vi "Example png string to imaq image.vi"() -> ()   [LabVIEW 2020]
uses:
  <vilib>/vision/Image Controls.llb/IMAQ Image.ctl
  <vilib>/wsapi/NI_WebServices.lvlib
  <vilib>/vision/NI_Vision_Development_Module.lvlib
panel:
  out "Image 2":T1(plugin-control)
  out "error out 2":errorcluster
  in  "error in (no error)":errorcluster
  out "Image Out":T1
  in  "File Path":path
  out "Image":T1(plugin-control)
  in  "String":string
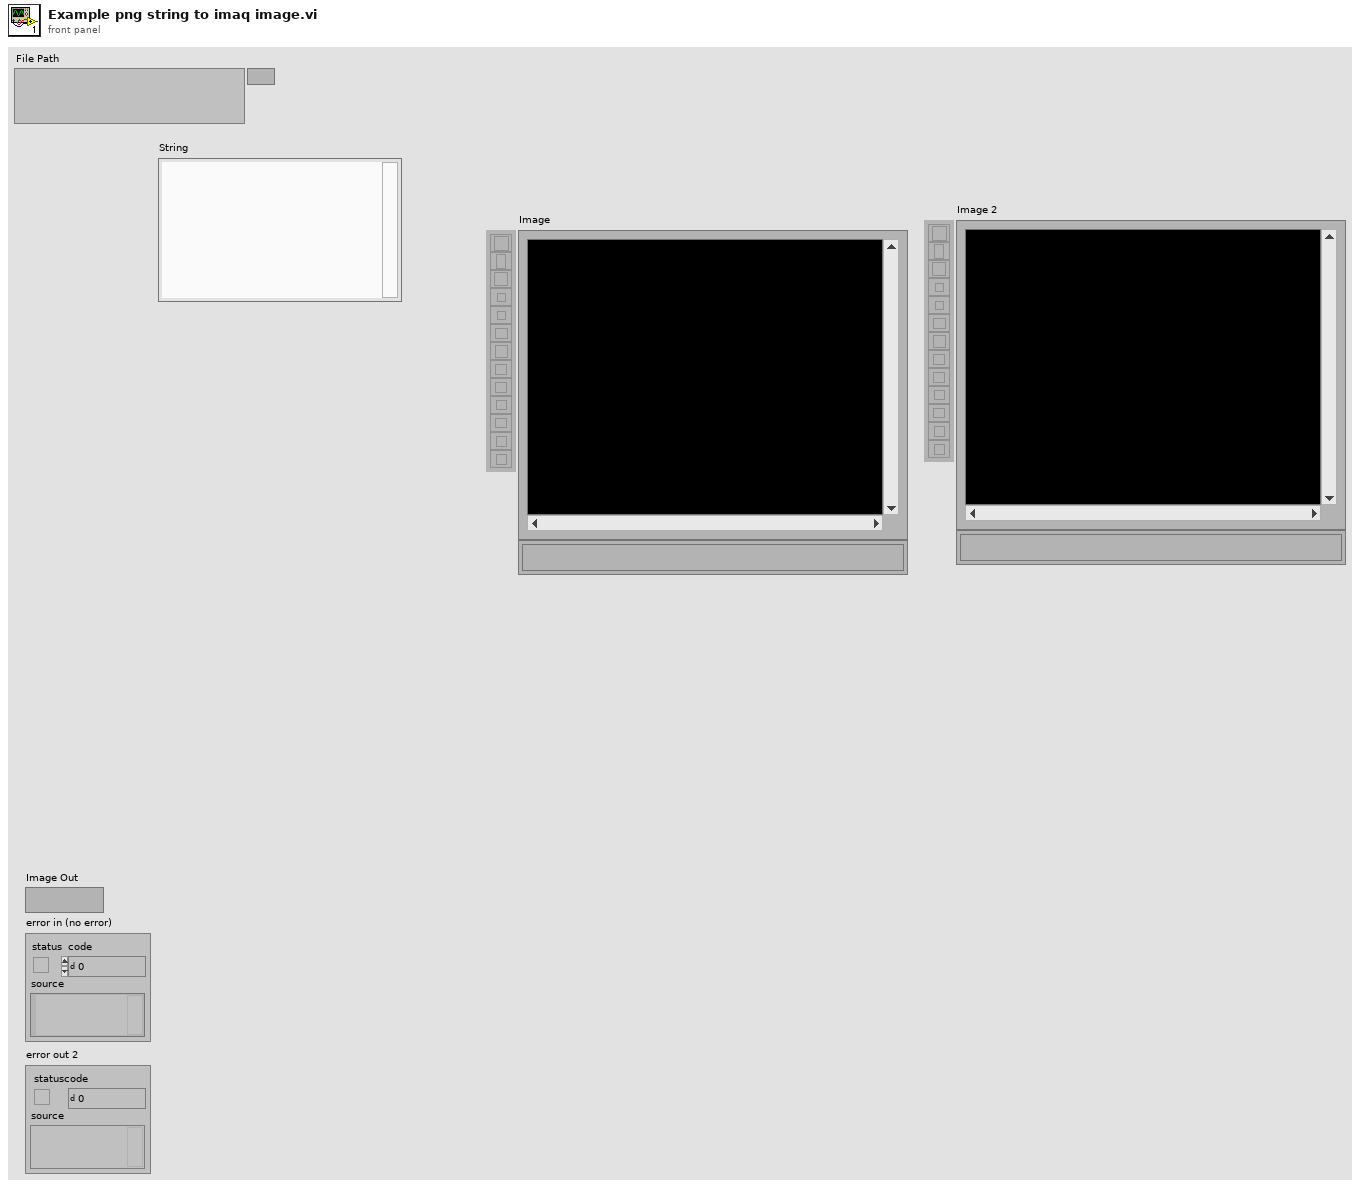
[diagram p1: front panel]
types:
  T1 = typedef "IMAQ Image.ctl" = refnum<image>
  T2 = typedef "Image Type" = u32
  T3 = typedef "imagedata.ctl" = cluster{"image type":i32, "image depth":i32, "image":u8[], "mask":u8[], "colors":u32[], "Rectangle":cluster{"left":i16, "top":i16, "right":i16, "bottom":i16}}
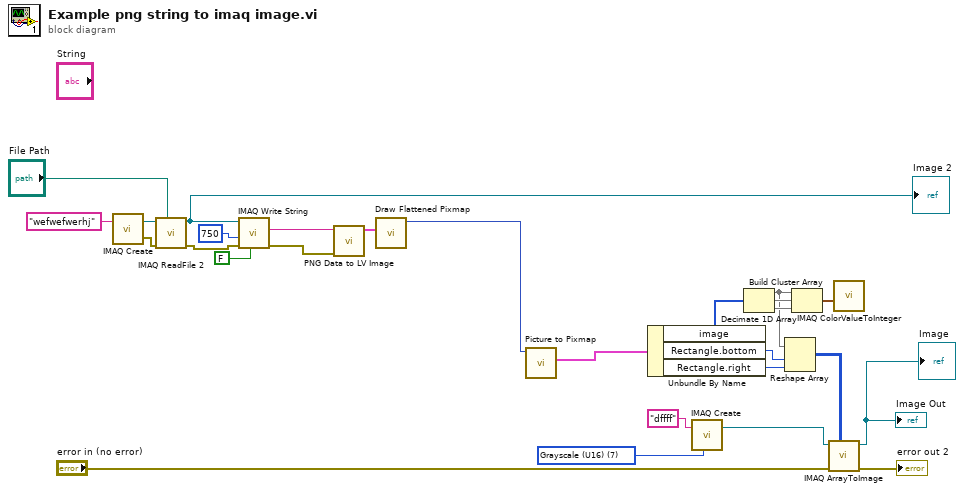
[diagram p0: block diagram]
diagram:
  w13 = T2 7 items=["Grayscale (U8)", "Grayscale (I16)", "Grayscale (SGL)", "Complex (CSG)", "RGB (U32)", "HSL (U32)", "RGB (U64)", "Grayscale (U16)"] ("Image Type")
  n1 = call "IMAQ Create"("Image Name"="wefwefwerhj") -> ("New Image"=w25:T1, "error out"=w5:errorcluster)  [unwired: 4 in]
  n2 = call "IMAQ ReadFile 2"("File Path"="File Path", "error in (no error)"=w5, "Image"=w25) -> ("error out"=w4:errorcluster, "Image Out"=w8:T1)  [unwired: 4 in, 3 out]
  "Image 2" <- w8
  n3 = call-poly "IMAQ Write String"("Use bit depth? (false)"=FALSE, "error in (no error)"=w4, "Image Quality"=u32 750, "Image"=w8) -> ("error out"=w3:errorcluster, "FileString"=w6:string)  [unwired: 5 in, 1 out]
  n4 = call <vilib>:"PNG Data to LV Image.vi"("error in (no error)"=w3, "png data"=w6) -> ("image data"=w20:T3)  [unwired: 8 in, 1 out]
  n5 = call <vilib>:"Draw Flattened Pixmap.vi"("image data"=w20) -> ("new picture"=w24:picture)  [unwired: 8 in]
  n6 = call <vilib>:"Picture to Pixmap.vi"("picture"=w24) -> ("image data"=w23:T3)  [unwired: 9 in, 1 out]
  n7 = Unbundle By Name(w23) -> ("image"=w9:u8[], "Rectangle.bottom"=w22:i16, "Rectangle.right"=w21:i16)
  n8 = call "IMAQ Create"("Image Name"="dffff", "Image Type"=w13) -> ("New Image"=w14:T1)  [unwired: 3 in, 1 out]
  n9 = Decimate 1D Array(w9) -> (w2:u8[], w12:u8[], w11:u8[])
  n10 = Reshape Array(w2, w22, w21) -> (w19:u8[][])
  n11 = Build Cluster Array(w2, w12, w11) -> (w10:cluster{u8, u8, u8}[])
  n12 = call "IMAQ ArrayToImage"("Image Pixels (U16)"=w19, "error in (no error)"="error in (no error)", "Image"=w14) -> ("error out"=→"error out 2":errorcluster, "Image Out"=→"Image" →"Image Out":T1)  [unwired: 7 in]
  n13 = call "IMAQ ColorValueToInteger"("1D Color value array"=w10) -> ()  [unwired: 4 in, 4 out]
